vi "VISA Get Session.vi"(8 "error in (no error)":errorcluster, 11 "Instrument.lvclass in":refnum<class "Instrument.lvclass">) -> (0 "error out":errorcluster, 1 "GPIB string":string="0", 2 "VISA Resource Name":refnum<visa-resource-name>, 3 "Instrument.lvclass out":refnum<class "Instrument.lvclass">)   [LabVIEW 2017, in "Instrument.lvclass"]
doc: "(Dynamic) Access the VISA session constructed for this Instrument. (Use this to send commands to the Instrument.) Override this method if the Instrument has communication idiosyncrasies."
uses:
  Instrument.lvclass
  Instrument.lvclass/Instrument.ctl
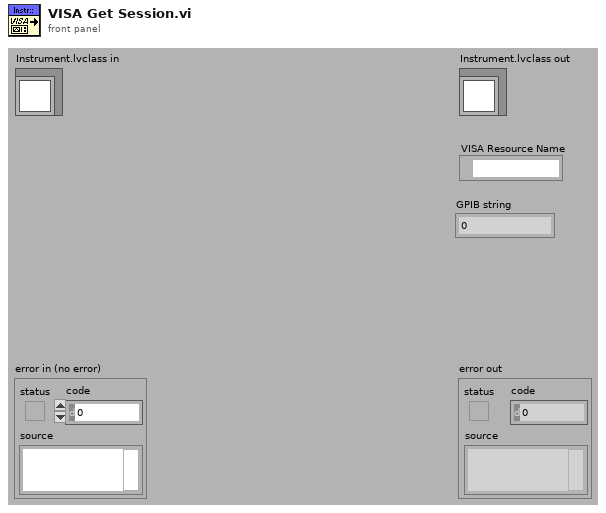
[diagram p1: front panel]
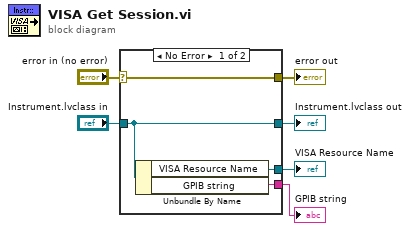
[diagram p0: block diagram]
diagram:
  n1 = case shown="No Error" "error in (no error)" {
    selector: "error in (no error)" -> [w10 w11]
    tunnel: [w10 w11] -> w5
    tunnel: [w9 w12] -> w3
    tunnel: "Instrument.lvclass in" -> [w9 w12]
    tunnel: [w8 _] -> w2
    tunnel: [w7 _] -> w1
    frame No Error {
      n2 = Unbundle By Name(w9) -> ("VISA Resource Name"=w8:refnum<visa-resource-name>, "GPIB string"=w7:string)
    }
    frame Error {
    }
  }
  "error out" <- w5
  "Instrument.lvclass out" <- w3
  "VISA Resource Name" <- w2
  "GPIB string" <- w1
